vi "氨氮流程步骤.vi"() -> ()   [LabVIEW 2016]
panel:
  out "步骤时间/秒":T1={"步骤1时间"=2, "步骤2时间"=4, "步骤3时间"=2, "步骤4时间"=5, "步骤5时间"=6, "步骤6时间"=3, "步骤7时间"=4, "步骤8时间"=7, "步骤9时间"=8, "步骤10时间"=6}
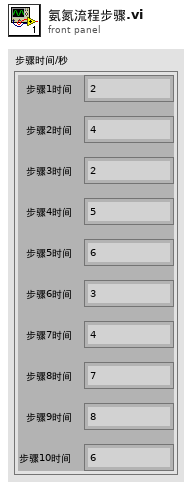
[diagram p1: front panel]
types:
  T1 = cluster{"步骤1时间":i32, "步骤2时间":i32, "步骤3时间":i32, "步骤4时间":i32, "步骤5时间":i32, "步骤6时间":i32, "步骤7时间":i32, "步骤8时间":i32, "步骤9时间":i32, "步骤10时间":i32}
  T2 = enum16{"步骤1", "步骤2", "步骤3", "步骤4", "步骤5", "步骤6", "步骤7", "步骤8", "步骤9", "步骤10"}
  T3 = cluster{"因子编码":u32, "单位":u16, "标样参考值":sgl, "水样数据时间":timestamp, "水样实测值":sgl, "水样数据标识":string, "标样数据时间":timestamp, "标样实测值":sgl, "标样数据标识":string, "空白数据时间":timestamp, "空白实测值":sgl, "空白数据标识":string, "零点核查数据时间":timestamp, "零点核查实测值":sgl, "零点核查数据标识":string, "跨度核查数据时间":timestamp, "跨度核查实测值":sgl, "跨度核查数据标识":string, "加标回收数据时间":timestamp, "加标回收实测值":sgl, "加标回收数据标识":string, "平行样数据时间":timestamp, "平行样实测值":sgl, "平行样数据标识":string}
  T4 = cluster{"系统时间":timestamp, "工作状态":u16, "测量模式":u16, "告警代码":enum16{"无告警", "缺试剂告警", "缺水样告警", "缺蒸馏水告警", "缺标液告警", "仪表漏液告警", "标定异常告警", "超量程告警", "加热异常", "低试剂预警", "超上限告警", "超下限告警", "仪表内部其他异常", "滴定异常告警", "电极异常告警", "量程切换告警", "参数设置告警", "PH电极电位异常", "电导率电极异常", "浊度光度异常", "溶解氧电极异常", "溶解氧光强异常", "温度异常告警", "PH异常告警", "溶解氧异常告警", "电导率异常告警", "浊度异常告警", "叶绿素异常告警", "藻密度异常告警", "蓝绿藻异常告警", "ORP异常告警", "氨氮异常告警", "清洁刷异常告警", "SD卡异常告警", "蓝牙异常告警", "Wifi异常告警", "流程异常告警"}, "故障代码":enum16{"无故障", "电机故障", "温度故障", "通讯故障", "滴定故障"}, "日志代码":u16, "软件版本":u16, "F0":sgl, "F1":sgl, "F2":sgl, "F3":sgl, "T":sgl, "H":sgl, "id":u16, "flowid":u16, "量程":u16}
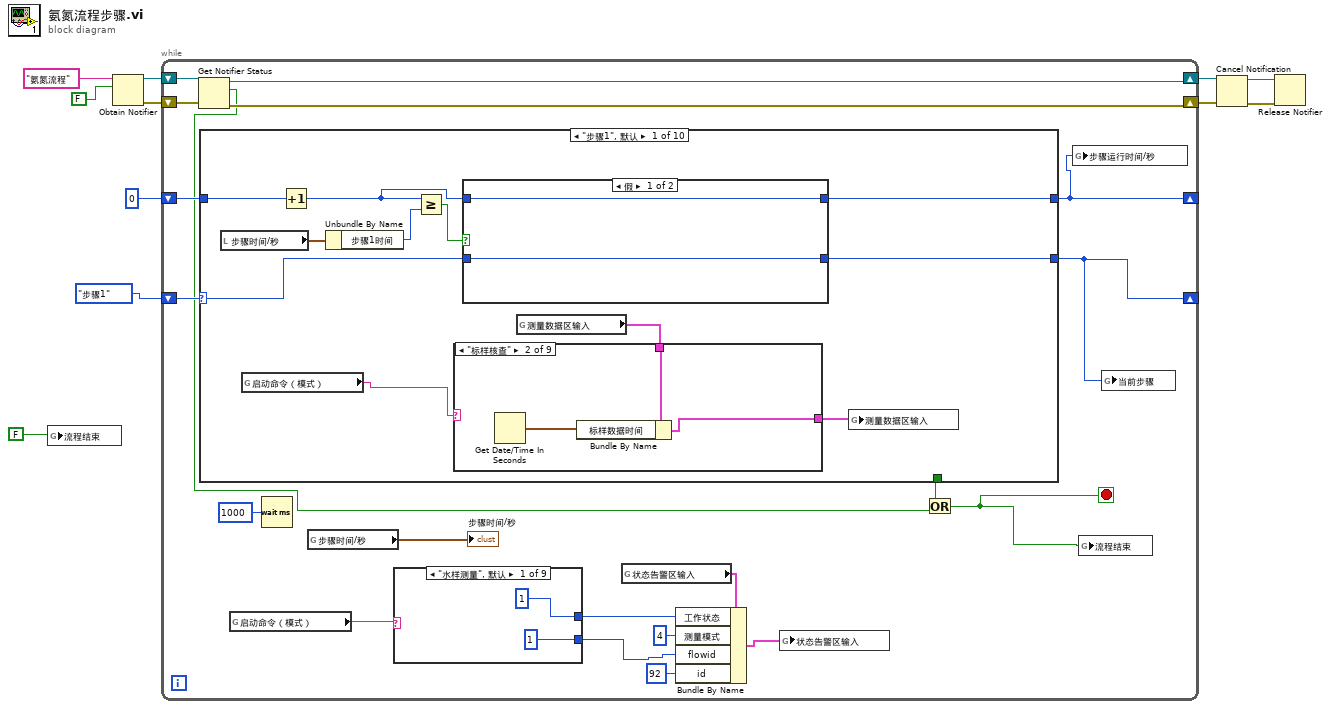
[diagram p0: block diagram]
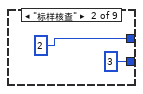
[diagram p2: hidden frame]
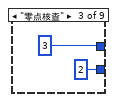
[diagram p3: hidden frame]
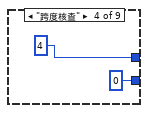
[diagram p4: hidden frame]
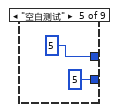
[diagram p5: hidden frame]
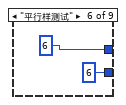
[diagram p6: hidden frame]
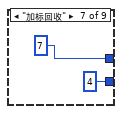
[diagram p7: hidden frame]
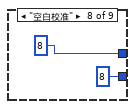
[diagram p8: hidden frame]
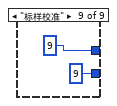
[diagram p9: hidden frame]
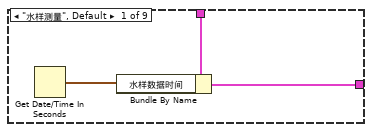
[diagram p10: hidden frame]
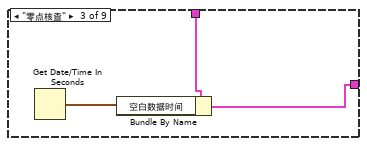
[diagram p11: hidden frame]
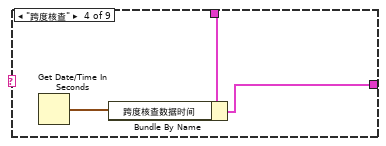
[diagram p12: hidden frame]
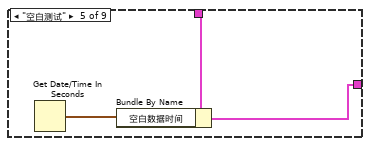
[diagram p13: hidden frame]
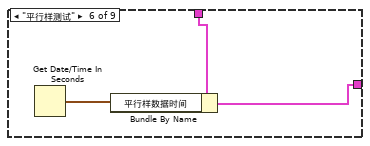
[diagram p14: hidden frame]
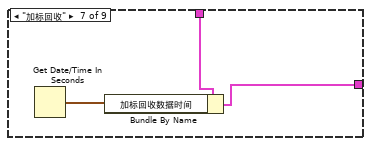
[diagram p15: hidden frame]
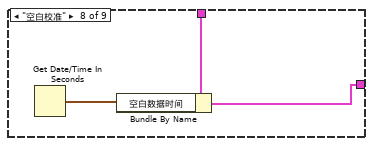
[diagram p16: hidden frame]
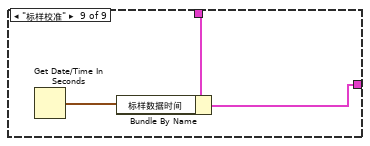
[diagram p17: hidden frame]
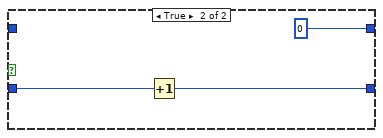
[diagram p18: hidden frame]
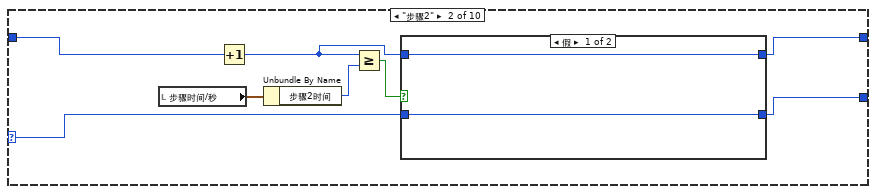
[diagram p19: hidden frame]
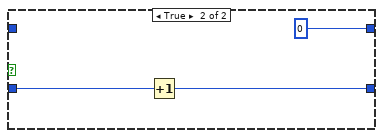
[diagram p20: hidden frame]
diagram:
  n1 = global write "氨氮全局.vi" "流程结束"(FALSE ("流程结束")) -> ()
  n2 = Obtain Notifier(name (unnamed)="氨氮流程" ("名称（未命名）"), notification data type=FALSE) -> (notifier out=w7:refnum<notifier>, error out=w6:errorcluster)  [unwired: 2 in, 1 out]
  n3 = while {
    shift-right: [w18] -> _
    shift-left: T2."步骤1" -> [w31]
    shift-right: [w17] -> _
    shift-left: 0 -> [w29]
    shift-right: [w25] -> w3
    shift-left: w7 -> [w27]
    shift-right: [w24] -> w2
    shift-left: w6 -> [w26]
    stop <- w16 stop-if-true
    n4 = Get Notifier Status(notifier=w27, error in (no error)=w26) -> (notifier out=w25:refnum<notifier>, current notification=w23:bool, error out=w24:errorcluster)  [unwired: 2 out]
    n5 = case shown="\"步骤1\", 默认" w31 {
      selector: w31 -> [w54 w95 w108 w121 w134 w147 w160 w173 w186 w200]
      tunnel: [_ _ _ _ _ _ _ _ _ w197] -> w28
      tunnel: w29 -> [w60 w96 w109 w122 w135 w148 w161 w174 w187 w201]
      tunnel: [w56 w94 w107 w120 w133 w146 w159 w172 w185 w199] -> w17
      tunnel: [w53 w93 w106 w119 w132 w145 w158 w171 w184 w198] -> w18
      frame "步骤1", Default {
        n6 = local read "步骤时间/秒"() -> (w59:T1)
        n7 = global read "氨氮全局.vi" "启动命令（模式）"() -> (w50:string)
        n8 = Increment(x=w60) -> (x+1=w55:i32)
        n9 = Unbundle By Name(w59) -> ("步骤1时间"=w58:i32)
        n10 = Greater Or Equal?(x=w55, y=w58) -> (x >= y?=w57:bool)
        n11 = case shown="假" w57 {
          tunnel: [w89 0] -> w56
          tunnel: w55 -> [w89 _]
          tunnel: w54 -> [w88 w91]
          tunnel: [w88 w90] -> w53
          frame False {
          }
          frame True {
            n12 = Increment(x=w91) -> (x+1=w90:T2)
          }
        }
        n13 = global read "氨氮全局.vi" "测量数据区输入"() -> (w52:T3)
        n14 = case shown="\"标样核查\"" w50 {
          tunnel: w52 -> [w62 w65 w68 w71 w74 w77 w80 w83 w86]
          tunnel: [w61 w64 w67 w70 w73 w76 w79 w82 w85] -> w51
          frame "水样测量", Default {
            n15 = Get Date/Time In Seconds() -> (seconds since 1Jan1904=w63:timestamp)
            n16 = Bundle By Name(cluster=w62, "水样数据时间"=w63) -> (w61:T3)
          }
          frame "标样核查" {
            n17 = Get Date/Time In Seconds() -> (seconds since 1Jan1904=w66:timestamp)
            n18 = Bundle By Name(cluster=w65, "标样数据时间"=w66) -> (w64:T3)
          }
          frame "零点核查" {
            n19 = Get Date/Time In Seconds() -> (seconds since 1Jan1904=w69:timestamp)
            n20 = Bundle By Name(cluster=w68, "空白数据时间"=w69) -> (w67:T3)
          }
          frame "跨度核查" {
            n21 = Get Date/Time In Seconds() -> (seconds since 1Jan1904=w72:timestamp)
            n22 = Bundle By Name(cluster=w71, "跨度核查数据时间"=w72) -> (w70:T3)
          }
          frame "空白测试" {
            n23 = Get Date/Time In Seconds() -> (seconds since 1Jan1904=w75:timestamp)
            n24 = Bundle By Name(cluster=w74, "空白数据时间"=w75) -> (w73:T3)
          }
          frame "平行样测试" {
            n25 = Get Date/Time In Seconds() -> (seconds since 1Jan1904=w78:timestamp)
            n26 = Bundle By Name(cluster=w77, "平行样数据时间"=w78) -> (w76:T3)
          }
          frame "加标回收" {
            n27 = Get Date/Time In Seconds() -> (seconds since 1Jan1904=w81:timestamp)
            n28 = Bundle By Name(cluster=w80, "加标回收数据时间"=w81) -> (w79:T3)
          }
          frame "空白校准" {
            n29 = Get Date/Time In Seconds() -> (seconds since 1Jan1904=w84:timestamp)
            n30 = Bundle By Name(cluster=w83, "空白数据时间"=w84) -> (w82:T3)
          }
          frame "标样校准" {
            n31 = Get Date/Time In Seconds() -> (seconds since 1Jan1904=w87:timestamp)
            n32 = Bundle By Name(cluster=w86, "标样数据时间"=w87) -> (w85:T3)
          }
        }
        n33 = global write "氨氮全局.vi" "测量数据区输入"(w51) -> ()
      }
      frame "步骤2" {
        n34 = local read "步骤时间/秒"() -> (w100:T1)
        n35 = Increment(x=w96) -> (x+1=w97:i32)
        n36 = Unbundle By Name(w100) -> ("步骤2时间"=w99:i32)
        n37 = Greater Or Equal?(x=w97, y=w99) -> (x >= y?=w98:bool)
        n38 = case shown="假" w98 {
          tunnel: [w102 0] -> w94
          tunnel: w97 -> [w102 _]
          tunnel: w95 -> [w101 w104]
          tunnel: [w101 w103] -> w93
          frame False {
          }
          frame True {
            n39 = Increment(x=w104) -> (x+1=w103:T2)
          }
        }
      }
      frame "步骤3" {
        n40 = local read "步骤时间/秒"() -> (w113:T1)
        n41 = Increment(x=w109) -> (x+1=w110:i32)
        n42 = Unbundle By Name(w113) -> ("步骤3时间"=w112:i32)
        n43 = Greater Or Equal?(x=w110, y=w112) -> (x >= y?=w111:bool)
        n44 = case shown="假" w111 {
          tunnel: [w115 0] -> w107
          tunnel: w110 -> [w115 _]
          tunnel: w108 -> [w114 w117]
          tunnel: [w114 w116] -> w106
          frame False {
          }
          frame True {
            n45 = Increment(x=w117) -> (x+1=w116:T2)
          }
        }
      }
      frame "步骤4" {
        n46 = local read "步骤时间/秒"() -> (w126:T1)
        n47 = Increment(x=w122) -> (x+1=w123:i32)
        n48 = Unbundle By Name(w126) -> ("步骤4时间"=w125:i32)
        n49 = Greater Or Equal?(x=w123, y=w125) -> (x >= y?=w124:bool)
        n50 = case shown="假" w124 {
          tunnel: [w128 0] -> w120
          tunnel: w123 -> [w128 _]
          tunnel: w121 -> [w127 w130]
          tunnel: [w127 w129] -> w119
          frame False {
          }
          frame True {
            n51 = Increment(x=w130) -> (x+1=w129:T2)
          }
        }
      }
      frame "步骤5" {
        n52 = local read "步骤时间/秒"() -> (w139:T1)
        n53 = Increment(x=w135) -> (x+1=w136:i32)
        n54 = Unbundle By Name(w139) -> ("步骤5时间"=w138:i32)
        n55 = Greater Or Equal?(x=w136, y=w138) -> (x >= y?=w137:bool)
        n56 = case shown="假" w137 {
          tunnel: [w141 0] -> w133
          tunnel: w136 -> [w141 _]
          tunnel: w134 -> [w140 w143]
          tunnel: [w140 w142] -> w132
          frame False {
          }
          frame True {
            n57 = Increment(x=w143) -> (x+1=w142:T2)
          }
        }
      }
      frame "步骤6" {
        n58 = local read "步骤时间/秒"() -> (w152:T1)
        n59 = Increment(x=w148) -> (x+1=w149:i32)
        n60 = Unbundle By Name(w152) -> ("步骤6时间"=w151:i32)
        n61 = Greater Or Equal?(x=w149, y=w151) -> (x >= y?=w150:bool)
        n62 = case shown="假" w150 {
          tunnel: [w154 0] -> w146
          tunnel: w149 -> [w154 _]
          tunnel: w147 -> [w153 w156]
          tunnel: [w153 w155] -> w145
          frame False {
          }
          frame True {
            n63 = Increment(x=w156) -> (x+1=w155:T2)
          }
        }
      }
      frame "步骤7" {
        n64 = local read "步骤时间/秒"() -> (w165:T1)
        n65 = Increment(x=w161) -> (x+1=w162:i32)
        n66 = Unbundle By Name(w165) -> ("步骤7时间"=w164:i32)
        n67 = Greater Or Equal?(x=w162, y=w164) -> (x >= y?=w163:bool)
        n68 = case shown="假" w163 {
          tunnel: [w167 0] -> w159
          tunnel: w162 -> [w167 _]
          tunnel: w160 -> [w166 w169]
          tunnel: [w166 w168] -> w158
          frame False {
          }
          frame True {
            n69 = Increment(x=w169) -> (x+1=w168:T2)
          }
        }
      }
      frame "步骤8" {
        n70 = local read "步骤时间/秒"() -> (w178:T1)
        n71 = Increment(x=w174) -> (x+1=w175:i32)
        n72 = Unbundle By Name(w178) -> ("步骤8时间"=w177:i32)
        n73 = Greater Or Equal?(x=w175, y=w177) -> (x >= y?=w176:bool)
        n74 = case shown="假" w176 {
          tunnel: [w180 0] -> w172
          tunnel: w175 -> [w180 _]
          tunnel: w173 -> [w179 w182]
          tunnel: [w179 w181] -> w171
          frame False {
          }
          frame True {
            n75 = Increment(x=w182) -> (x+1=w181:T2)
          }
        }
      }
      frame "步骤9" {
        n76 = local read "步骤时间/秒"() -> (w191:T1)
        n77 = Increment(x=w187) -> (x+1=w188:i32)
        n78 = Unbundle By Name(w191) -> ("步骤9时间"=w190:i32)
        n79 = Greater Or Equal?(x=w188, y=w190) -> (x >= y?=w189:bool)
        n80 = case shown="假" w189 {
          tunnel: [w193 0] -> w185
          tunnel: w188 -> [w193 _]
          tunnel: w186 -> [w192 w195]
          tunnel: [w192 w194] -> w184
          frame False {
          }
          frame True {
            n81 = Increment(x=w195) -> (x+1=w194:T2)
          }
        }
      }
      frame "步骤10" {
        n82 = local read "步骤时间/秒"() -> (w205:T1)
        n83 = Increment(x=w201) -> (x+1=w202:i32)
        n84 = Unbundle By Name(w205) -> ("步骤10时间"=w204:i32)
        n85 = Greater Or Equal?(x=w202, y=w204) -> (x >= y?=w203:bool)
        n86 = case shown="真" w203 {
          tunnel: [w207 0] -> w199
          tunnel: w202 -> [w207 _]
          tunnel: w200 -> [w206 w210]
          tunnel: [w206 w209] -> w198
          tunnel: [_ TRUE] -> w197
          frame False {
          }
          frame True {
            n87 = Increment(x=w210) -> (x+1=w209:T2)
          }
        }
      }
    }
    n88 = global read "氨氮全局.vi" "启动命令（模式）"() -> (w12:string)
    n89 = Wait (ms)(milliseconds to wait=u32 1000 ("等待时间（毫秒）")) -> ()  [unwired: 1 out]
    n90 = global read "氨氮全局.vi" "步骤时间/秒"() -> (→"步骤时间/秒":T1)
    n91 = case shown="\"水样测量\", 默认" w12 {
      tunnel: [u16 1 ("工作状态") u16 2 ("工作状态") u16 3 ("工作状态") u16 4 ("工作状态") u16 5 ("工作状态") u16 6 ("工作状态") u16 7 ("工作状态") u16 8 ("工作状态") u16 9 ("工作状态")] -> w21
      tunnel: [u16 1 ("工作状态") u16 3 ("工作状态") u16 2 ("工作状态") u16 0 ("工作状态") u16 5 ("工作状态") u16 6 ("工作状态") u16 4 ("工作状态") u16 8 ("工作状态") u16 9 ("工作状态")] -> w19
      frame "水样测量", Default {
      }
      frame "标样核查" {
      }
      frame "零点核查" {
      }
      frame "跨度核查" {
      }
      frame "空白测试" {
      }
      frame "平行样测试" {
      }
      frame "加标回收" {
      }
      frame "空白校准" {
      }
      frame "标样校准" {
      }
    }
    n92 = global read "氨氮全局.vi" "状态告警区输入"() -> (w14:T4)
    n93 = Bundle By Name(cluster=w14, "工作状态"=w21, "测量模式"=u16 4, "flowid"=w19, "id"=u16 92) -> (w15:T4)
    n94 = global write "氨氮全局.vi" "状态告警区输入"(w15) -> ()
    n95 = Or(x=w28, y=w23) -> (x .or. y?=w16:bool)
    n96 = global write "氨氮全局.vi" "步骤运行时间/秒"(w17) -> ()
    n97 = global write "氨氮全局.vi" "流程结束"(w16) -> ()
    n98 = global write "氨氮全局.vi" "当前步骤"(w18) -> ()
  }
  n99 = Cancel Notification(0:w3, 3:w2) -> (8:w5:refnum<notifier>, 11:w4:errorcluster)  [unwired: 1 out]
  n100 = Release Notifier(notifier=w5, error in (no error)=w4) -> ()  [unwired: 1 in, 3 out]
